vi "RpeakDetector(subVI).vi"(0 "EDA":dbl[](array[numeric]), 1 "Vstupní signál":waveform(dbl)) -> (2 "Max èas":dbl, 3 "Min èas":dbl, 4 "Signál s peaky a EDA":waveform(dbl)[](array[waveform]), 5 "BPM":i32, 6 "XY-HRV":cluster{dbl[], dbl[]})   [LabVIEW 2026]
uses:
  <vilib>/Analysis/3filter.llb/Filter Passband Type.ctl
  <vilib>/Analysis/baseanly.llb/Mean (DBL).vi
  <vilib>/Analysis/3filter.llb/Butterworth Filter (DBL).vi
  <vilib>/Waveform/WDTOps.llb/WDT Waveform to XY Pairs DBL.vi
  <vilib>/Analysis/NI_AAL_SigProc.lvlib
  <vilib>/Analysis/NI_AALBase.lvlib
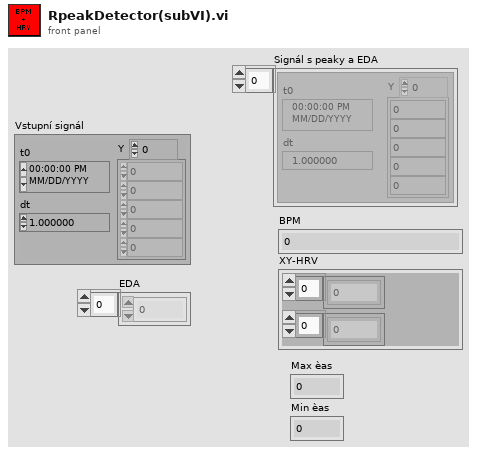
[diagram p1: front panel]
types:
  T1 = typedef "NI_AALBase.lvlib/Filter Passband Type.ctl" = enum32{"Lowpass", "Highpass", "Bandpass", "Bandstop"}
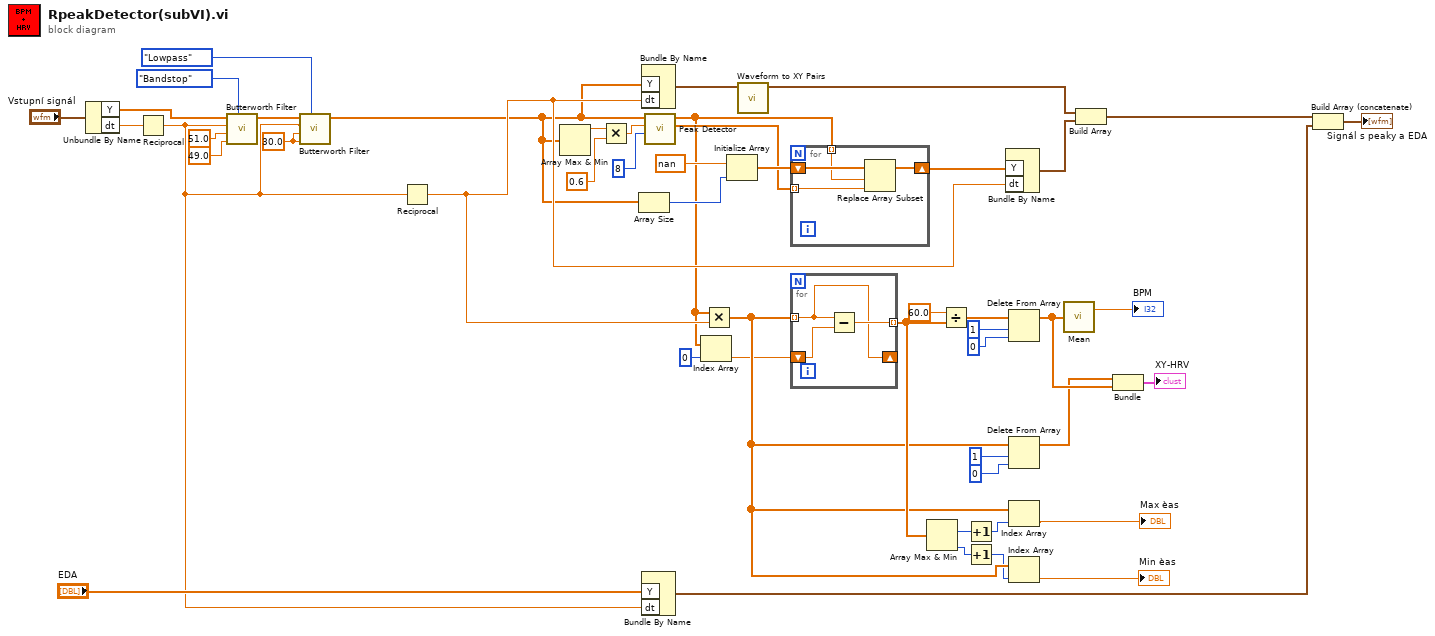
[diagram p0: block diagram]
diagram:
  w19 = 30.0 ("high cutoff freq: fh")
  n1 = Unbundle By Name("Vstupní signál") -> ("Y"=w21:dbl[], "dt"=w20:dbl)
  n2 = Reciprocal(x=w20) -> (1/x=w16:dbl)
  n3 = call-poly <vilib>:"Butterworth Filter.vi"("filter type"=Filter_Passband_Type."Bandstop", "low cutoff freq: fl"=49.0, "high cutoff freq: fh"=51.0, "sampling freq: fs"=w16, "X"=w21) -> ("Filtered X"=w27:dbl[])  [unwired: 3 in, 1 out]
  n4 = call-poly <vilib>:"Butterworth Filter.vi"("filter type"=Filter_Passband_Type."Lowpass", "low cutoff freq: fl"=w19, "high cutoff freq: fh"=w19, "sampling freq: fs"=w16, "X"=w27) -> ("Filtered X"=w26:dbl[])  [unwired: 3 in, 1 out]
  n5 = Reciprocal(x=w16) -> (1/x=w31:dbl)
  n6 = Array Max & Min(array=w26) -> (max value=w40:dbl)  [unwired: 3 out]
  n7 = Multiply(x=w40, y=0.6) -> (x*y=w38:dbl)
  n8 = Array Size(array=w26) -> (size(s)=w46:i32)
  n9 = Bundle By Name("Y"=w26, "dt"=w31) -> (w48:waveform(dbl))  [unwired: 1 in]
  n10 = Bundle By Name("Y"="EDA", "dt"=w16) -> (w14:waveform(dbl))  [unwired: 1 in]
  n11 = call <vilib>:"Peak Detector.vi"("width"=8, "threshold"=w38, "X"=w26) -> ("Amplitudes"=w43:dbl[], "Locations"=w5:dbl[])  [unwired: 4 in, 3 out]
  n12 = Index Array(array=w5, index=0) -> (element=w4:dbl)
  n13 = Multiply(x=w5, y=w31) -> (x*y=w7:dbl[])
  n14 = Initialize Array(nan, w46) -> (w44:dbl[])
  n15 = call-poly <vilib>:"Waveform to XY Pairs.vi"("waveform in"=w48) -> ("waveform out"=w47:waveform(dbl))  [unwired: 8 in, 2 out]
  n16 = for {
    tunnel: w5 -> [w52] mode=indexing
    tunnel: w43 -> [w51] mode=indexing
    shift-right: [w50] -> w42
    shift-left: w44 -> [w53]
    n17 = Replace Array Subset(array=w53, new element=w51, index=w52) -> (w50:dbl[])
  }
  n18 = for {
    shift-right: [w54] -> _
    shift-left: w4 -> [w56]
    tunnel: w7 -> [w54] mode=indexing
    tunnel: [w55] -> w11 mode=indexing
    n19 = Subtract(x=w54, y=w56) -> (x-y=w55:dbl)
  }
  n20 = Array Max & Min(array=w11) -> (max index (indices)=w10:i32, min index (indices)=w9:i32)  [unwired: 2 out]
  n21 = Divide(x=60.0, y=w11) -> (x/y=w35:dbl[])
  n22 = Increment(x=w10) -> (x+1=w8:i32)
  n23 = Increment(x=w9) -> (x+1=w6:i32)
  n24 = Bundle By Name("Y"=w42, "dt"=w31) -> (w41:waveform(dbl))  [unwired: 1 in]
  n25 = Delete From Array(array=w35, length=1, index=0) -> (array with subset deleted=w32:dbl[])  [unwired: 1 out]
  n26 = Delete From Array(array=w7, length=1, index=0) -> (array with subset deleted=w24:dbl[])  [unwired: 1 out]
  n27 = Index Array(array=w7, index=w8) -> (element=→"Max èas":dbl)
  n28 = Index Array(array=w7, index=w6) -> (element=→"Min èas":dbl)
  n29 = call-poly <vilib>:"Mean.vi"("X"=w32) -> ("mean"=→"BPM":dbl)  [unwired: 1 out]
  n30 = Build Array(w47, w41) -> (w15:waveform(dbl)[])
  n31 = Bundle(w24, w32) -> (→"XY-HRV":cluster{dbl[], dbl[]})  [unwired: 1 in]
  n32 = Build Array (concatenate)(w15, w14) -> (→"Signál s peaky a EDA":waveform(dbl)[])
